vi "Create Plugins.vi"(8 "error in (no error)":errorcluster, 9 "components directory":path, 10 "Plugin Configurations":T1[](array[typedef]) {"Transfer Groups"."Transfers"."channels"."buffer offset" format="%d bytes"}, 11 "Framework in":refnum<class "Framework.lvclass">) -> (0 "error out":errorcluster, 1 "Inline Plugins":refnum<class "Plugin.lvclass">[](array[class]), 2 "Async Plugins":refnum<class "Plugin.lvclass">[](array[class]), 3 "Framework out":refnum<class "Framework.lvclass">)   [LabVIEW 2017, in "DSF Core.lvlib" / "Framework.lvclass"]
uses:
  Framework.lvclass
  DSF Configuration API/Public/Controls/DSF Engine Plugin Configuration.ctl
  DSF Configuration API/Public/Controls/DSF Timing Info.ctl
  DSF Configuration API/Public/Controls/DSF Engine Transfer Group Configuration.ctl
  DSF Configuration API/Public/Controls/DSF Direction.ctl
  DSF Configuration API/Public/Controls/DSF Engine Transfer Configuration.ctl
  DSF Configuration API/Public/Controls/DSF Byte Order.ctl
  DSF Configuration API/Public/Controls/DSF Engine Channel Configuration.ctl
  DSF Configuration API/Public/Controls/DSF Data Type.ctl
  DSF Configuration API/Public/Controls/DSF Settings Info.ctl
  Plugin/Plugin.lvclass
  Framework.lvclass/Framework.ctl
  Shared/Constants/Default Components Directory.vi
  Component Loader/Component Loader.lvclass
  DSF Core.lvlib
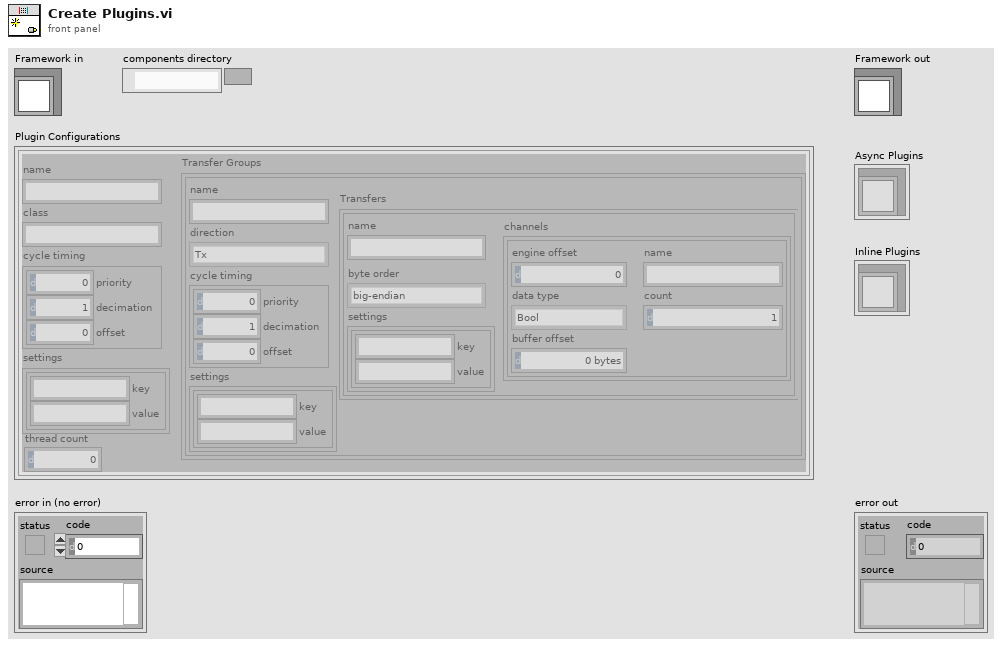
[diagram p1: front panel]
types:
  T1 = typedef "DSF Core.lvlib/DSF Engine Plugin Configuration.ctl" = cluster{"name":string, "class":string, "cycle timing":T2, "Transfer Groups":T3[], "settings":T9, "thread count":i32}
  T2 = typedef "DSF Core.lvlib/DSF Timing Info.ctl" = cluster{"priority":u64, "decimation":u64, "offset":u64}
  T3 = typedef "DSF Core.lvlib/DSF Engine Transfer Group Configuration.ctl" = cluster{"name":string, "direction":T4, "cycle timing":T2, "Transfers":T5[], "settings":T9}
  T4 = typedef "DSF Core.lvlib/DSF Direction.ctl" = enum8{"Tx", "Rx"}
  T5 = typedef "DSF Core.lvlib/DSF Engine Transfer Configuration.ctl" = cluster{"name":string, "byte order":T6, "channels":T7[], "settings":T9}
  T6 = typedef "DSF Core.lvlib/DSF Byte Order.ctl" = enum8{"big-endian", "little-endian"}
  T7 = typedef "DSF Core.lvlib/DSF Engine Channel Configuration.ctl" = cluster{"engine offset":u64, "name":string, "data type":T8, "count":u64, "buffer offset":u64}
  T8 = typedef "DSF Core.lvlib/DSF Data Type.ctl" = enum8{"Bool", "SGL", "DBL", "I8", "I16", "I32", "I64", "U8", "U16", "U32", "U64"}
  T9 = typedef "DSF Core.lvlib/DSF Settings Info.ctl" = cluster{"key":string, "value":string}[]
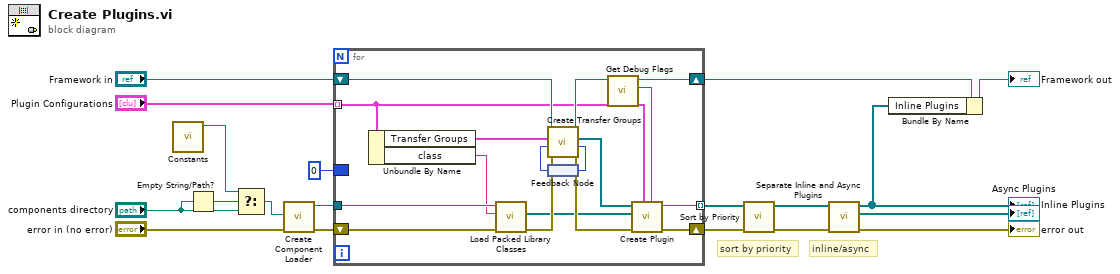
[diagram p0: block diagram]
diagram:
  # "inline/async"
  # "sort by priority"
  n1 = call-poly "Constants.vi"() -> ("Default Components Directory"=w8:path)  [unwired: 11 in]
  n2 = Empty String/Path?(string/path="components directory") -> (empty?=w11:bool)
  n3 = Select(t=w8, s=w11, f="components directory") -> (s? t:f=w9:path)
  n4 = call "Create Component Loader.vi"("error in (no error)"="error in (no error)", "components directory"=w9) -> ("error out"=w16:errorcluster, "Component Loader out"=w17:refnum<class "Component Loader.lvclass">)  [unwired: 8 in]
  n5 = for {
    shift-right: [w34] -> w19
    shift-left: w16 -> [w27]
    shift-right: [w30] -> w3
    shift-left: "Framework in" -> [w33]
    tunnel: "Plugin Configurations" -> [w23] mode=indexing
    tunnel: [w32] -> w18 mode=indexing
    tunnel: w17 -> [w29]
    border: 0 ("ending id") -> [_]
    n6 = Unbundle By Name(w23) -> ("Transfer Groups"=w26:T3[], "class"=w25:string)
    n7 = call "Load Packed Library Classes.vi"("error in (no error)"=w27, "packed library name"=w25, "Component Loader in"=w29) -> ("error out"=w35:errorcluster, "objects"=w22:refnum<class>[])  [unwired: 6 in, 1 out]
    n8 = feedback #1() -> (w20:i32)
    n9 = call "Create Transfer Groups.vi"("error in (no error)"=w35, "starting id"=w20, "Transfer Group Configurations"=w26, "Framework in"=w33) -> ("error out"=w36:errorcluster, "ending id"=w21:i32, "Transfer Groups"=w24:refnum<class "Transfer Group.lvclass">[], "Framework out"=w31:refnum<class "Framework.lvclass">)  [unwired: 4 in]
    n10 = feedback-in #1(w21) -> ()
    n11 = call "Get Debug Flags.vi"("Framework in"=w31) -> ("Debug Flags"=w28:refnum<class "Debug Flags.lvclass">, "Framework out"=w30:refnum<class "Framework.lvclass">)  [unwired: 9 in]
    n12 = call "Create Plugin.vi"("Debug Flags"=w28, "Plugin Configuration"=w23, "error in (no error)"=w36, "component classes"=w22, "Transfer Groups"=w24) -> ("error out"=w34:errorcluster, "Plugin out"=w32:refnum<class "Plugin.lvclass">)  [unwired: 5 in]
  }
  n13 = call "Sort by Priority.vi"("error in (no error)"=w19, "Plugins in"=w18) -> ("error out"=w7:errorcluster, "Plugins out"=w5:refnum<class "Plugin.lvclass">[])  [unwired: 8 in]
  n14 = call "Separate Inline and Async Plugins.vi"("error in (no error)"=w7, "Plugins"=w5) -> ("error out"=→"error out":errorcluster, "Async Plugins"=→"Async Plugins":refnum<class "Plugin.lvclass">[], "Inline Plugins"=w1:refnum<class "Plugin.lvclass">[])  [unwired: 7 in]
  "Inline Plugins" <- w1
  n15 = Bundle By Name(cluster=w3, "Inline Plugins"=w1) -> (→"Framework out":refnum<class "Framework.lvclass">)
